vi "DiJian_2.vi"(8 "error in":errorcluster, 9 "地检2相位":i32, 11 "VISA资源名称":refnum<visa-resource-name>) -> (0 "错误输出":errorcluster, 1 "地检2相位输出":i32, 3 "VISA资源名称输出":refnum<visa-resource-name>)   [LabVIEW 2012]
uses:
  <vilib>/GPower/VIRegister/Library/Convert/ToDBL.vi
  <vilib>/GPower/VIRegister/Library/Convert/ToU16.vi
  <vilib>/GPower/VIRegister/Library/SubVIs/FindRegisterData.vi
  <vilib>/GPower/VIRegister/Library/SubVIs/ReadSub.vi
  <vilib>/GPower/VIRegister/Library/QManager/GetRegisterData.vi
  <vilib>/GPower/Error/Library/SetError.vi
  <vilib>/GPower/Error/Library/FilterCodes.vi
  <vilib>/GPower/Error/Library/Filter/FilterMulti.vi
  <vilib>/GPower/VIRegister/Library/QManager/QManagerAction.vi
  <vilib>/GPower/Error/Library/ErrorType.vi
  <vilib>/GPower/Error/Library/SplitAppended.vi
  <vilib>/GPower/Error/Library/SubVIs/ExplanationToError.vi
  <vilib>/GPower/VIRegister/Library/QManager/GetQName.vi
  <vilib>/GPower/VIRegister/Library/QManager/StartQManager.vi
  <vilib>/Utility/error.llb/Trim Whitespace.vi
  <vilib>/dlg_ctls.llb/Space Constant.vi
  <vilib>/Utility/error.llb/Error Code Database.vi
  <vilib>/GPower/Error/Library/SubVIs/SetStatus.vi
  <vilib>/GPower/Error/Library/AppendErrors.vi
  <vilib>/GPower/Error/Library/Append/AppendSingle.vi
  com/TONGXUN/write32.vi
  <vilib>/GPower/VIRegister/VIRegister.lvlib
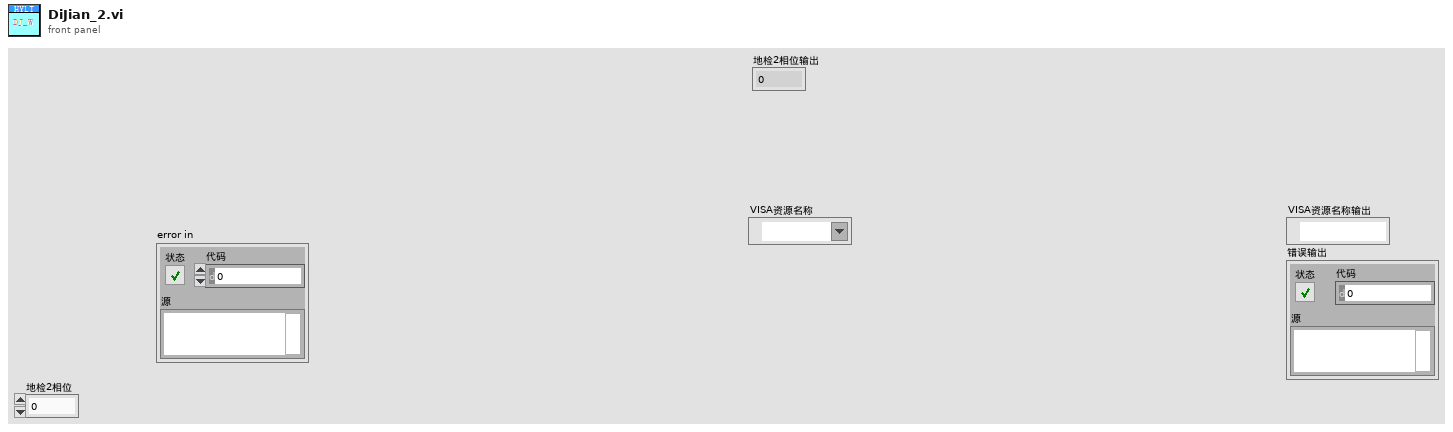
[diagram p1: front panel]
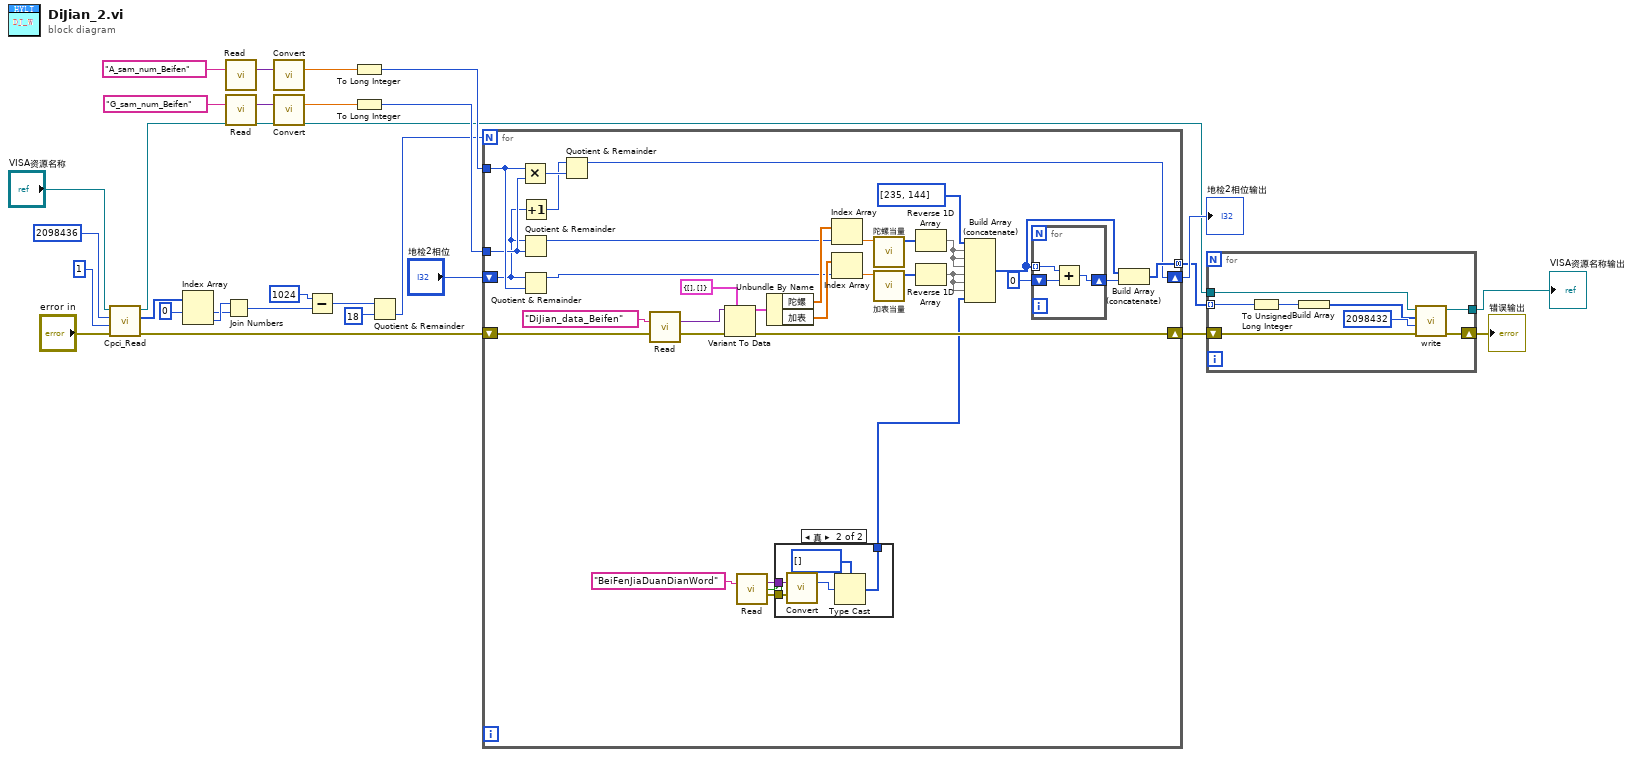
[diagram p0: block diagram]
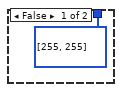
[diagram p2: hidden frame]
diagram:
  n1 = call "Cpci_Read.vi"("错误输入（无错误）"="error in", "u32_len"=1, "基地址"=u32 2098436, "VISA资源名称"="VISA资源名称") -> ("错误输出"=w1:errorcluster, "U8"=w9:u8[], "VISA资源名称输出"=w3:refnum<visa-resource-name>)  [unwired: 5 in]
  n2 = Index Array(array=w9, index #1=0 ("索引")) -> (element #1=w6:u8, element #2=w7:u8)  [unwired: 1 in]
  n3 = Join Numbers(hi=w7, lo=w6) -> ((hi.lo)=w12:u16)
  n4 = call <vilib>:"Read.vi"("Register name"="A_sam_num_Beifen") -> ("Register value"=w24:variant)  [unwired: 11 in, 3 out]
  n5 = call <vilib>:"Read.vi"("Register name"="G_sam_num_Beifen") -> ("Register value"=w21:variant)  [unwired: 11 in, 3 out]
  n6 = call-poly <vilib>:"Convert.vi"("Register value in"=w24) -> ("Register value out"=w25:dbl)  [unwired: 13 in, 1 out]
  n7 = call-poly <vilib>:"Convert.vi"("Register value in"=w21) -> ("Register value out"=w20:dbl)  [unwired: 13 in, 1 out]
  n8 = Subtract(x=u16 1024, y=w12) -> (x-y=w14:u16)
  n9 = To Long Integer(number=w25) -> (32bit integer=w22:i32)
  n10 = To Long Integer(number=w20) -> (32bit integer=w18:i32)
  n11 = Quotient & Remainder(x=w14, y=u16 18) -> (floor(x/y)=w5:u16)  [unwired: 1 out]
  n12 = for {
    N: w5 -> [_]
    tunnel: [w53] -> w4 mode=concatenating
    shift-right: [w52] -> w2
    shift-left: w1 -> [w51]
    shift-right: [w37] -> w16
    shift-left: "地检2相位" -> [w35]
    tunnel: w22 -> [w40]
    tunnel: w18 -> [w39]
    n13 = Multiply(x=w40, y=w39) -> (x*y=w38:i32)
    n14 = Increment(x=w35) -> (x+1=w36:i32)
    n15 = Quotient & Remainder(x=w35, y=w39) -> (x-y*floor(x/y)=w42:i32)  [unwired: 1 out]
    n16 = Quotient & Remainder(x=w35, y=w40) -> (x-y*floor(x/y)=w41:i32)  [unwired: 1 out]
    n17 = Quotient & Remainder(x=w36, y=w38) -> (x-y*floor(x/y)=w37:i32)  [unwired: 1 out]
    n18 = call <vilib>:"Read.vi"("Register name"="DiJian_data_Beifen", "Error in"=w51) -> ("Register value"=w59:variant, "Error out"=w55:errorcluster)  [unwired: 10 in, 2 out]
    n19 = Variant To Data(error in=w55, type=cluster{"陀螺":dbl[], "加表":dbl[]} {"陀螺"=[], "加表"=[]} ("输入簇"), Variant=w59) -> (data=w60:cluster{"陀螺":dbl[], "加表":dbl[]}, error out=w52:errorcluster)
    n20 = call <vilib>:"Read.vi"("Register name"="BeiFenJiaDuanDianWord") -> ("Register value"=w32:variant, "Register value read?"=w31:bool, "Error out"=w33:errorcluster)  [unwired: 11 in, 1 out]
    n21 = Unbundle By Name(w60) -> ("陀螺"=w61:dbl[], "加表"=w62:dbl[])
    n22 = case shown="真" w31 {
      tunnel: w33 -> [_ w68]
      tunnel: w32 -> [_ w67]
      tunnel: [u8[] [255, 255] ("反转的数组") w65] -> w30
      frame False {
      }
      frame True {
        n23 = call-poly <vilib>:"Convert.vi"("Register value in"=w67, "Error in"=w68) -> ("Register value out"=w66:u16)  [unwired: 12 in, 1 out]
        n24 = Type Cast(type=u8[] [] ("反转的数组"), x=w66) -> (*(type *) &x=w65:u8[])
      }
    }
    n25 = Index Array(array=w61, index=w42) -> (element=w49:dbl)
    n26 = Index Array(array=w62, index=w41) -> (element=w47:dbl)
    n27 = call "陀螺当量.vi"("x"=w49) -> ("子数组"=w48:u8[])  [unwired: 10 in]
    n28 = call "加表当量.vi"("x"=w47) -> ("子数组"=w46:u8[])  [unwired: 10 in]
    n29 = Reverse 1D Array(array=w48) -> (reversed array=w44:u8[])
    n30 = Reverse 1D Array(array=w46) -> (reversed array=w43:u8[])
    n31 = Build Array (concatenate)(u8[] [235, 144] ("数组"), w44, w44, w44, w43, w43, w43, w30) -> (w45:u8[])
    n32 = for {
      tunnel: w45 -> [w71] mode=indexing
      shift-right: [w69] -> w56
      shift-left: u8 0 ("y") -> [w70]
      n33 = Add(x=w71, y=w70) -> (x+y=w69:u8)
    }
    n34 = Build Array (concatenate)(w45, w56) -> (w53:u8[])
  }
  "地检2相位输出" <- w16
  n35 = for {
    tunnel: w4 -> [w79] mode=indexing
    tunnel: w3 -> [w78]
    tunnel: [w77] -> w28
    shift-right: [w75] -> w26
    shift-left: w2 -> [w76]
    n36 = To Unsigned Long Integer(number=w79) -> (unsigned 32bit integer=w72:u32)
    n37 = Build Array(w72) -> (w73:u32[])
    n38 = call-poly "write.vi"("error out"=w76, "起始地址"=u32 2098432, "U32"=w73, "VISA资源名称输入"=w78) -> ("error out 2"=w75:errorcluster, "VISA资源名称输出"=w77:refnum<visa-resource-name>)  [unwired: 6 in]
  }
  "VISA资源名称输出" <- w28
  "错误输出" <- w26
